vi "sv_Nth Order Intermodulation Components.vi"(6 "include harmonics":bool, 7 "order":i32, 10 "f2":dbl format="%.2f", 11 "f1":dbl format="%.2f") -> (3 "Nth order intermodulation components":dbl[](array[numeric]) format="%.2f")   [LabVIEW 2017, in "SoundVib_Distortion.lvlib"]
uses:
  <vilib>/addons/Sound and Vibration/svt_Distortion/SoundVib_Distortion.lvlib
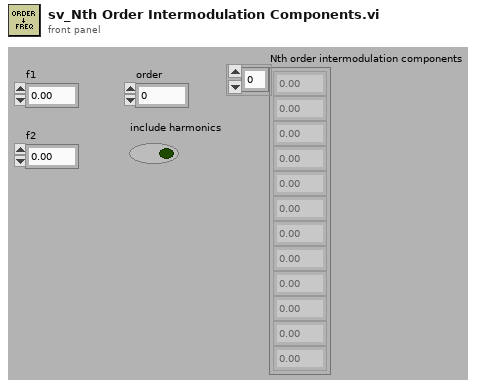
[diagram p1: front panel]
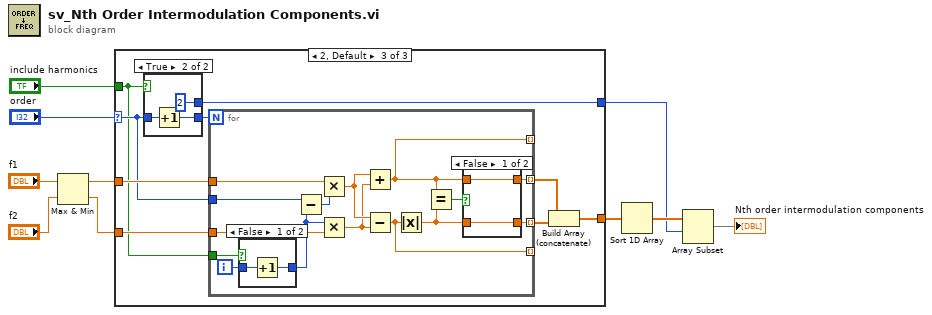
[diagram p0: block diagram]
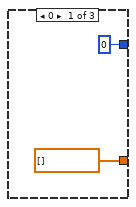
[diagram p2: hidden frame]
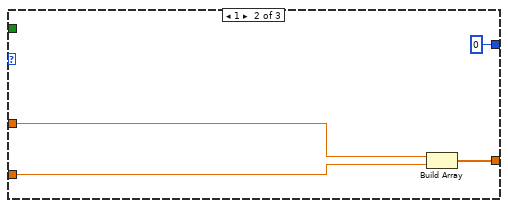
[diagram p3: hidden frame]
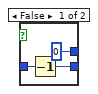
[diagram p4: hidden frame]
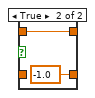
[diagram p6: hidden frame]
diagram:
  n1 = Max & Min(x="f1", y="f2") -> (max(x,y)=w4:dbl, min(x,y)=w3:dbl)
  n2 = case shown="2, Default" "order" {
    selector: "order" -> [_ _ w20]
    tunnel: [dbl[] [] w16 w25] -> w10
    tunnel: w4 -> [_ w15 w22]
    tunnel: w3 -> [_ w14 w21]
    tunnel: "include harmonics" -> [_ _ w18]
    tunnel: [0 ("Array Index") 0 ("Array Index") w17] -> w1
    frame 0 {
    }
    frame 1 {
      n3 = Build Array(w15, w14) -> (w16:dbl[])
    }
    frame 2, Default {
      n4 = case shown="True" w18 {
        tunnel: w20 -> [w28 w31]
        tunnel: [w27 w30] -> w19
        tunnel: [0 ("Array Index") 2 ("Array Index")] -> w17
        frame False {
          n5 = Decrement(x=w28) -> (x-1=w27:i32)
        }
        frame True {
          n6 = Increment(x=w31) -> (x+1=w30:i32)
        }
      }
      n7 = for {
        N: w19 -> [_]
        tunnel: w21 -> [w46]
        tunnel: w22 -> [w43]
        tunnel: [w38] -> w23 mode=indexing
        tunnel: [w37] -> w24 mode=indexing
        tunnel: w20 -> [w40]
        tunnel: [w32] -> _ mode=indexing
        tunnel: [w34] -> _ mode=indexing
        tunnel: w18 -> [w33]
        i -> [w45]
        n8 = case shown="False" w33 {
          tunnel: w45 -> [w48 w49]
          tunnel: [w47 w49] -> w35
          frame False {
            n9 = Increment(x=w48) -> (x+1=w47:i32)
          }
          frame True {
          }
        }
        n10 = Subtract(x=w40, y=w35) -> (x-y=w44:i32)
        n11 = Multiply(x=w43, y=w44) -> (x*y=w42:dbl)
        n12 = Multiply(x=w35, y=w46) -> (x*y=w41:dbl)
        n13 = Add(x=w42, y=w41) -> (x+y=w32:dbl)
        n14 = Subtract(x=w42, y=w41) -> (x-y=w34:dbl)
        n15 = Absolute Value(x=w34) -> (abs(x)=w36:dbl)
        n16 = Equal?(x=w32, y=w36) -> (x = y?=w39:bool)
        n17 = case shown="False" w39 {
          tunnel: [w51 w53] -> w38
          tunnel: w32 -> [w51 w53]
          tunnel: w36 -> [w50 _]
          tunnel: [w50 -1.0] -> w37
          frame False {
          }
          frame True {
          }
        }
      }
      n18 = Build Array (concatenate)(w23, w24) -> (w25:dbl[])
    }
  }
  n19 = Sort 1D Array(array=w10) -> (sorted array=w9:dbl[])
  n20 = Array Subset(array=w9, index=w1) -> (→"Nth order intermodulation components":dbl[])  [unwired: 1 in]
